vi "Synchronous generator.vi"() -> ()   [LabVIEW 2015]
panel:
  out "Waveform Graph":dynamicdata(graph)
  in  "Frequency":i32
  in  "Amplitude":i32
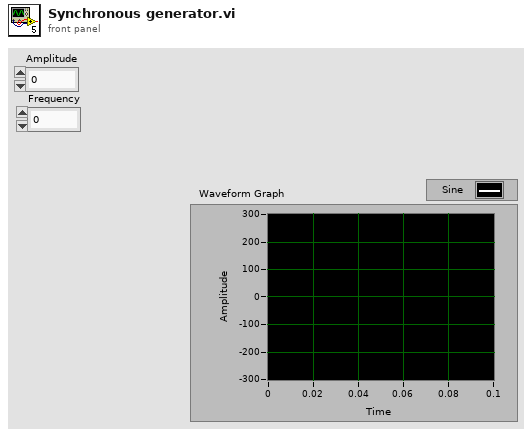
[diagram p1: front panel]
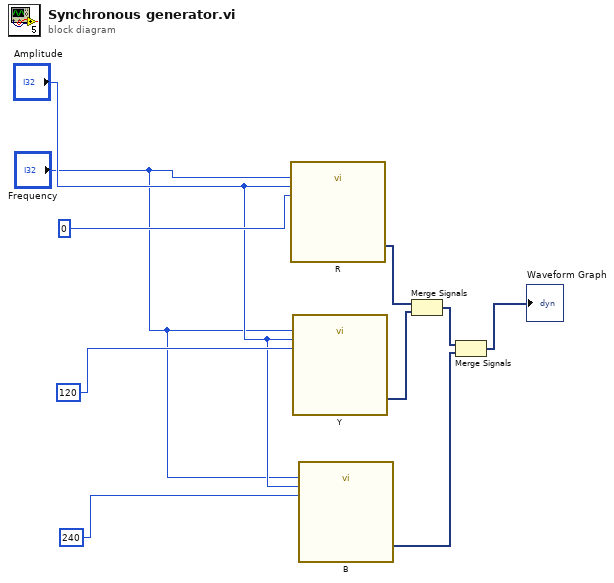
[diagram p0: block diagram]
diagram:
  n1 = call "R"("Frequency"="Frequency", "Amplitude"="Amplitude", "Phase"=0) -> ("Sine"=w5:dynamicdata)  [unwired: 11 in, 1 out]
  n2 = call "Y"("Frequency"="Frequency", "Amplitude"="Amplitude", "Phase"=120) -> ("Sine"=w4:dynamicdata)  [unwired: 11 in, 1 out]
  n3 = call "B"("Frequency"="Frequency", "Amplitude"="Amplitude", "Phase"=240) -> ("Sine"=w2:dynamicdata)  [unwired: 11 in, 1 out]
  n4 = Merge Signals(w5, w4) -> (w3:dynamicdata)
  n5 = Merge Signals(w3, w2) -> (→"Waveform Graph":dynamicdata)
